vi "WPI_JoystickGet.vi"(6 "Scaler":i8=127, 7 "JoystickDevRef":T1) -> (1 "Buttons":T4, 2 "Axes":T3, 3 "JoystickDevRef":T1)   [LabVIEW 2017]
doc: "Returns button and scaled axis information about a joystick that you specify. Use the GetAxis VI to return the scaled value of a specific axis of the joystick. Use the GetRawValue VI to return button and raw axis information about the joystick.\n\nThis software is licensed. Open the labview\\readme\\WPI Robotics Library Open Source License.txt file for more information."
uses:
  <vilib>/Rock Robotics/WPI/Joystick/WPI_JoystickDevRef.ctl
  <vilib>/Rock Robotics/WPI/Joystick/WPI_JoystickDeviceEnum.ctl
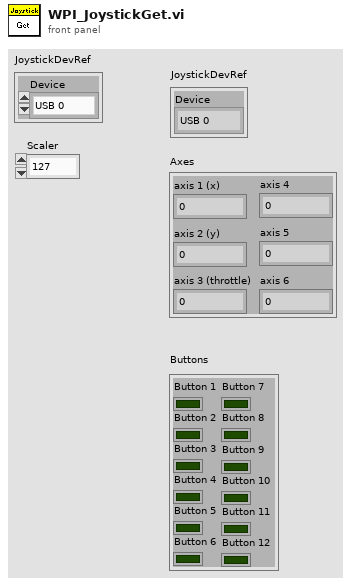
[diagram p1: front panel]
types:
  T1 = typedef "WPI_JoystickDevRef.ctl" = cluster{"Device":T2}
  T2 = typedef "WPI_JoystickDeviceEnum.ctl" = enum16{"USB 0", "USB 1", "USB 2", "USB 3", "USB 4", "USB 5"}
  T3 = cluster{"axis 1 (x)":dbl, "axis 2 (y)":dbl, "axis 3 (throttle)":dbl, "axis 4":dbl, "axis 5":dbl, "axis 6":dbl}
  T4 = cluster{"Button 1":bool, "Button 2":bool, "Button 3":bool, "Button 4":bool, "Button 5":bool, "Button 6":bool, "Button 7":bool, "Button 8":bool, "Button 9":bool, "Button 10":bool, "Button 11":bool, "Button 12":bool}
  T5 = cluster{"Axes[0]":dbl, "Axes[1]":dbl, "Axes[2]":dbl, "Axes[3]":dbl, "Axes[4]":dbl, "Axes[5]":dbl}
  T6 = cluster{"Buttons[0]":bool, "Buttons[1]":bool, "Buttons[2]":bool, "Buttons[3]":bool, "Buttons[4]":bool, "Buttons[5]":bool, "Buttons[6]":bool, "Buttons[7]":bool, "Buttons[8]":bool, "Buttons[9]":bool, "Buttons[10]":bool, "Buttons[11]":bool}
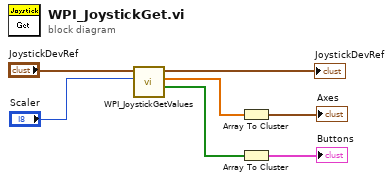
[diagram p0: block diagram]
diagram:
  n1 = call <vilib>:"WPI_JoystickGetValues.vi"("Scaler"="Scaler", "JoystickDevRef"="JoystickDevRef") -> ("Buttons"=w2:bool[], "Axes"=w4:dbl[], "JoystickDevRef"=→"JoystickDevRef":T1)  [unwired: 5 in, 2 out]
  n2 = Array To Cluster(array=w4) -> (cluster=→"Axes":T5)
  n3 = Array To Cluster(array=w2) -> (cluster=→"Buttons":T6)
